vi "CreateSettingsFolder.vi"(8 "error in (no error)":errorcluster) -> (0 "error out":errorcluster)   [LabVIEW 2015]
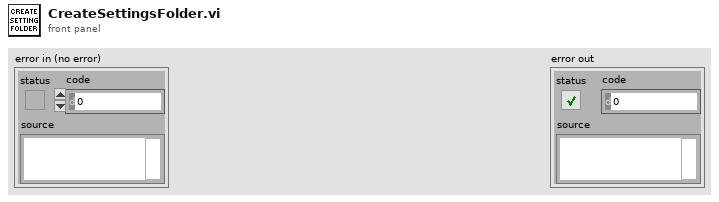
[diagram p1: front panel]
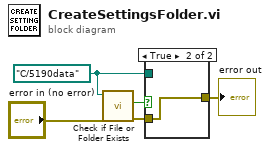
[diagram p0: block diagram]
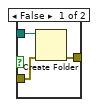
[diagram p2: hidden frame]
diagram:
  w5 = path "C:/5190data" ("path")
  n1 = call <vilib>:"Check if File or Folder Exists.vi"("error in (no error)"="error in (no error)", "path"=w5) -> ("error out"=w2:errorcluster, "file or folder exists?"=w4:bool)  [unwired: 7 in, 1 out]
  n2 = case shown="True" w4 {
    tunnel: w5 -> [w8 _]
    tunnel: w2 -> [w7 w9]
    tunnel: [w6 w9] -> w1
    frame False {
      n3 = Create Folder(path (use dialog)=w8, error in=w7) -> (error out=w6:errorcluster)  [unwired: 1 in, 2 out]
    }
    frame True {
    }
  }
  "error out" <- w1
